vi "34 GPS Time from Config (2017).vi"() -> (0 "GPS Lock":bool, 1 "Time":dbl)   [LabVIEW 2017]
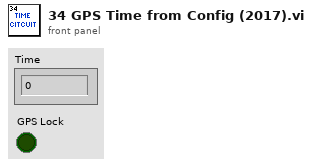
[diagram p1: front panel]
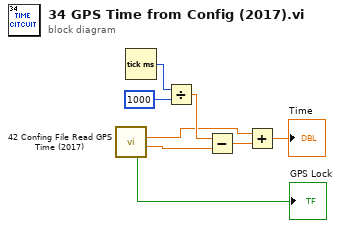
[diagram p0: block diagram]
diagram:
  n1 = call "42 Confing File Read GPS Time (2017).vi"() -> ("Labview Time"=w1:dbl, "GPS Lock"=→"GPS Lock":bool, "Tick Count"=w2:dbl)  [unwired: 10 in, 3 out]
  n2 = Tick Count (ms)() -> (millisecond timer value=w8:u32)
  n3 = Divide(x=w8, y=u32 1000) -> (x/y=w5:dbl)
  n4 = Subtract(x=w5, y=w2) -> (x-y=w6:dbl)
  n5 = Add(x=w1, y=w6) -> (x+y=→"Time":dbl)
